vi "loginDB.vi"(7 "error in (no error)":errorcluster caption="에러 입력(에러 없음)", 9 "Query":string, 10 "State":T1(ring)) -> (0 "error out":errorcluster caption="에러 출력", 3 "Result Set":string[][](table) caption="Result")   [LabVIEW 2019]
uses:
  <vilib>/drjdpowell/SQLite Library/SQL Connection/Connection.lvclass
  <vilib>/drjdpowell/SQLite Library/SQLite.lvlib
  <vilib>/drjdpowell/SQLite Library/SQL Connection/Execute SQL (Single String).vi
  <vilib>/drjdpowell/SQLite Library/SQL Connection/Execute SQL.vi
  <vilib>/drjdpowell/SQLite Library/SQL Connection/Open (path).vi
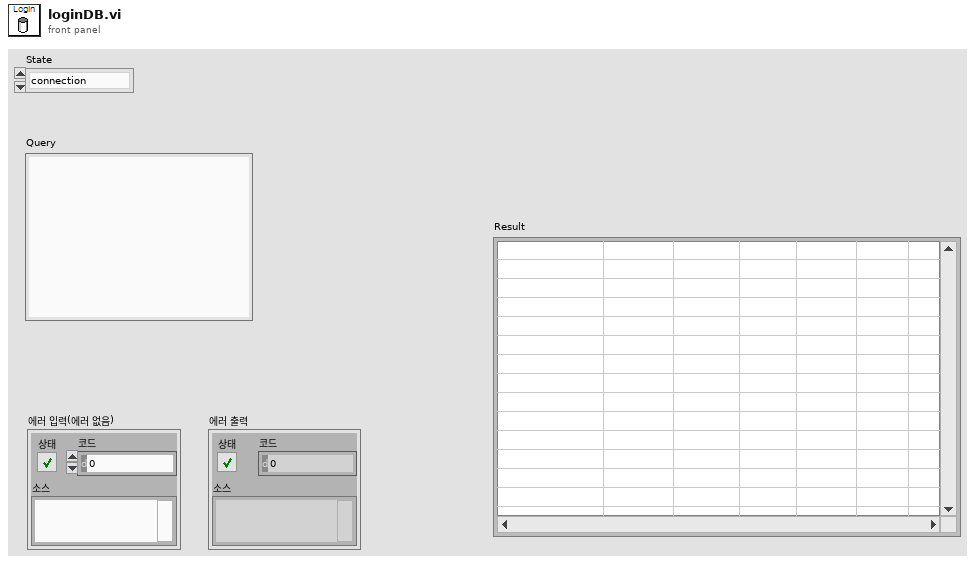
[diagram p1: front panel]
types:
  T1 = enum16{"connection", "create", "read", "update", "delete", "close"}
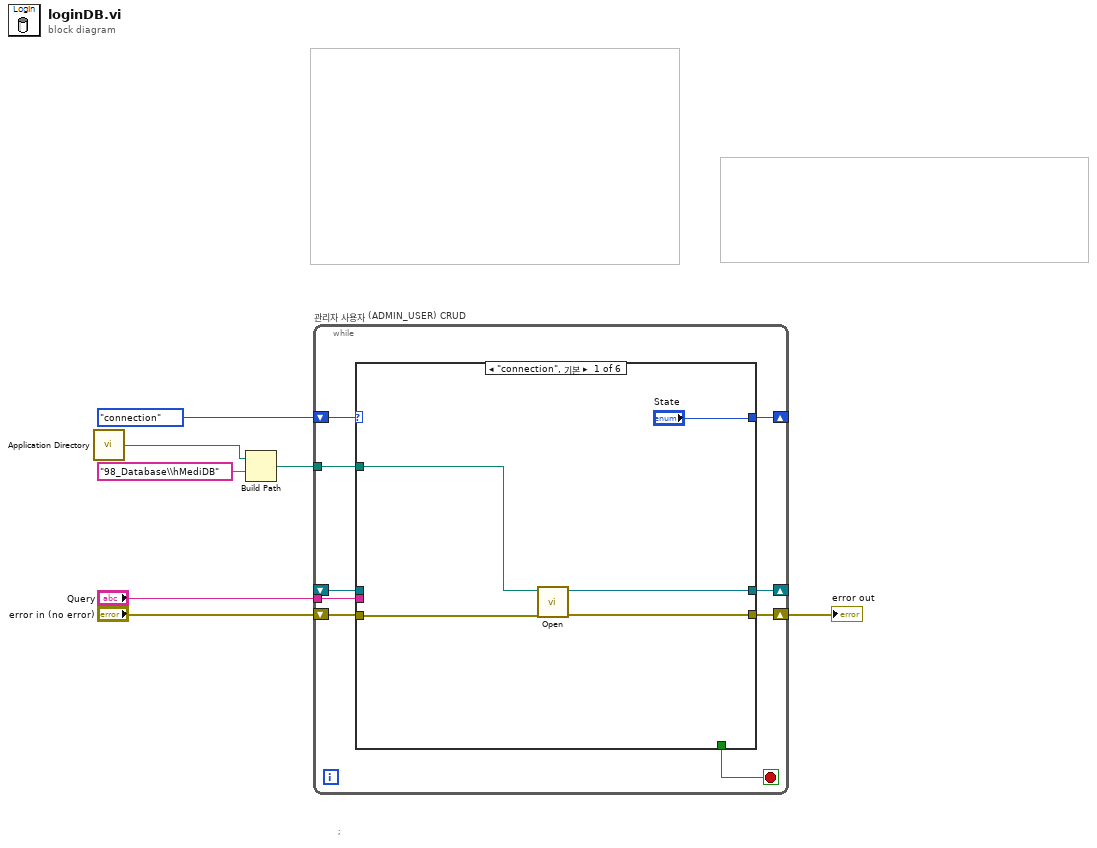
[diagram p0: block diagram]
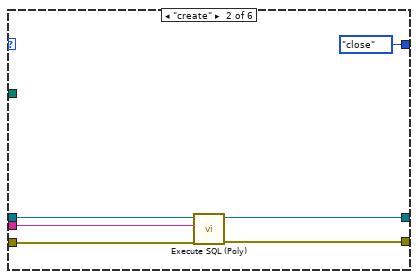
[diagram p2: hidden frame]
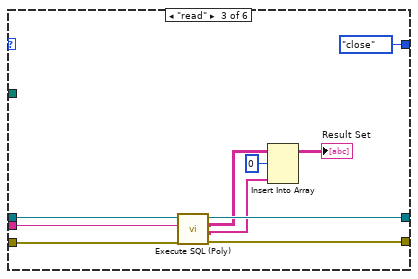
[diagram p3: hidden frame]
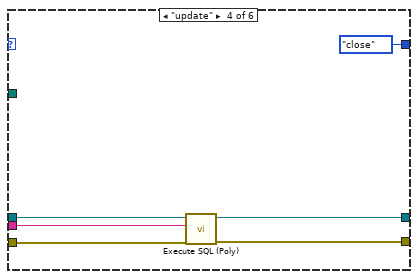
[diagram p4: hidden frame]
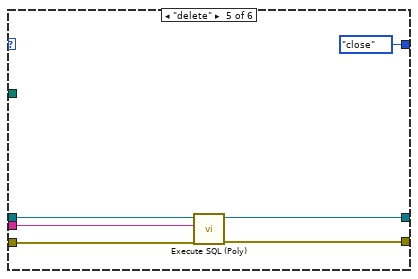
[diagram p5: hidden frame]
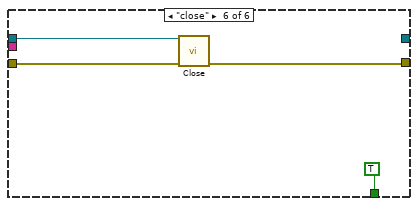
[diagram p6: hidden frame]
diagram:
  # ";"
  n1 = call <vilib>:"Application Directory.vi"() -> ("Application Directory"=w2:path)
  n2 = Build Path(base path=w2, name or relative path="98_Database\\hMediDB") -> (appended path=w1:path)
  n3 = while "관리자 사용자 (ADMIN_USER) CRUD" {
    shift-right: [w15] -> _
    shift-left: _ -> [w14]
    tunnel: w1 -> [w12]
    shift-right: [w11] -> _
    shift-left: T1."connection" ("State") -> [w16]
    shift-right: [w13] -> w4
    shift-left: "error in (no error)" -> [w9]
    tunnel: "Query" -> [w8]
    stop <- w10 stop-if-true
    n4 = case shown="\"connection\", 기본" w16 {
      tunnel: [w21 w25 w35 w41 w47 _] -> w15
      tunnel: w14 -> [_ w27 w37 w43 w49 w53]
      tunnel: [w20 w24 w34 w40 w46 w51] -> w13
      tunnel: w12 -> [w19 _ _ _ _ _]
      tunnel: w9 -> [w18 w26 w36 w42 w48 w52]
      tunnel: ["State" T1."close" ("State") T1."close" ("State") T1."close" ("State") T1."close" ("State") _] -> w11
      tunnel: [_ _ _ _ _ TRUE] -> w10
      tunnel: w8 -> [_ w22 w32 w38 w44 _]
      frame "connection", Default {
        n5 = call-poly <vilib>:"Open.vi"("error in (no error)"=w18, "db file"=w19) -> ("error out"=w20:errorcluster, "SQLite Connection"=w21:refnum<class "Connection.lvclass">)  [unwired: 8 in]
      }
      frame "create" {
        n6 = call-poly <vilib>:"Execute SQL (Poly).vi"("error in (no error)"=w26, "SQL"=w22, "SQLite Connection in"=w27) -> ("error out"=w24:errorcluster, "SQLite Connection"=w25:refnum<class "Connection.lvclass">)  [unwired: 6 in, 1 out]
      }
      frame "read" {
        n7 = call-poly <vilib>:"Execute SQL (Poly).vi"("error in (no error)"=w36, "SQL"=w32, "SQLite Connection in"=w37) -> ("error out"=w34:errorcluster, "Column Names"=w30:string[], "Result Set"=w31:string[][], "SQLite Connection"=w35:refnum<class "Connection.lvclass">)  [unwired: 5 in]
        n8 = Insert Into Array(array=w31, index (row)=0 ("인덱스 (행)"), new element=w30) -> (→"Result Set":string[][])  [unwired: 1 in]
      }
      frame "update" {
        n9 = call-poly <vilib>:"Execute SQL (Poly).vi"("error in (no error)"=w42, "SQL"=w38, "SQLite Connection in"=w43) -> ("error out"=w40:errorcluster, "SQLite Connection"=w41:refnum<class "Connection.lvclass">)  [unwired: 6 in, 1 out]
      }
      frame "delete" {
        n10 = call-poly <vilib>:"Execute SQL (Poly).vi"("error in (no error)"=w48, "SQL"=w44, "SQLite Connection in"=w49) -> ("error out"=w46:errorcluster, "SQLite Connection"=w47:refnum<class "Connection.lvclass">)  [unwired: 6 in, 1 out]
      }
      frame "close" {
        n11 = call-dynamic "Close.vi"("error in (no error)"=w52, "SQLite Connection in"=w53) -> ("error out"=w51:errorcluster)  [unwired: 9 in]
      }
    }
  }
  "error out" <- w4
